vi "gamedata.vi"(10 "set(T)/get(F) 2":bool, 11 "String 2":string) -> (0 "s? t:f":string)   [LabVIEW 2017]
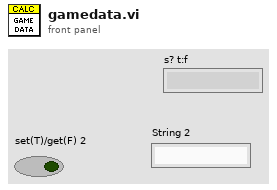
[diagram p1: front panel]
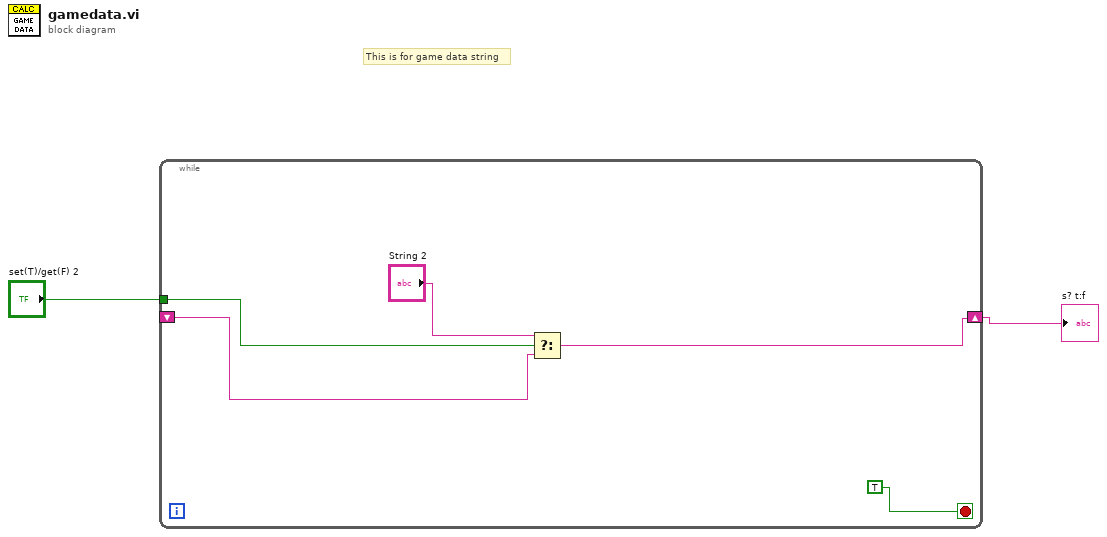
[diagram p0: block diagram]
diagram:
  # "This is for game data string"
  n1 = while {
    shift-right: [w5] -> w2
    shift-left: _ -> [w4]
    tunnel: "set(T)/get(F) 2" -> [w6]
    stop <- TRUE stop-if-true
    n2 = Select(t="String 2", s=w6, f=w4) -> (s? t:f=w5:string)
  }
  "s? t:f" <- w2
